vi "Calculator.vi"() -> ()   [LabVIEW 2015]
panel:
  out "Display":string
  out "Numeric 2":dbl
  out "Numeric":dbl format="%#_9g"
  out "Operator":string
  in  "N":dbl=1.0
  in  "Boolean":bool
  in  "stop":bool
  in  "8":bool
  in  "=":bool
  in  ".":bool
  in  "+":bool
  in  "3":bool
  in  "0":bool
  in  "Negative":bool
  in  "2":bool
  in  "1":bool
  in  "-":bool
  in  "6":bool
  in  "*":bool
  in  "9":bool
  in  "5":bool
  in  "4":bool
  in  "7":bool
  in  "\\":bool
  in  "C":bool
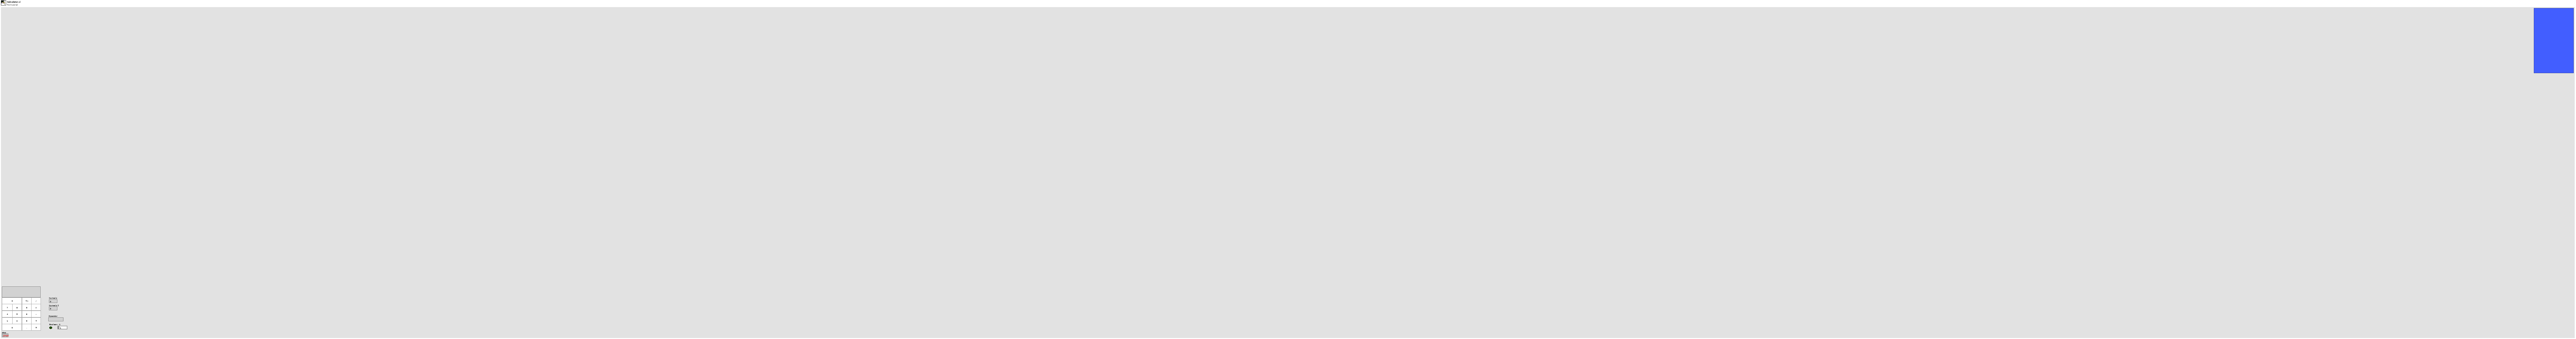
[diagram p1: front panel]
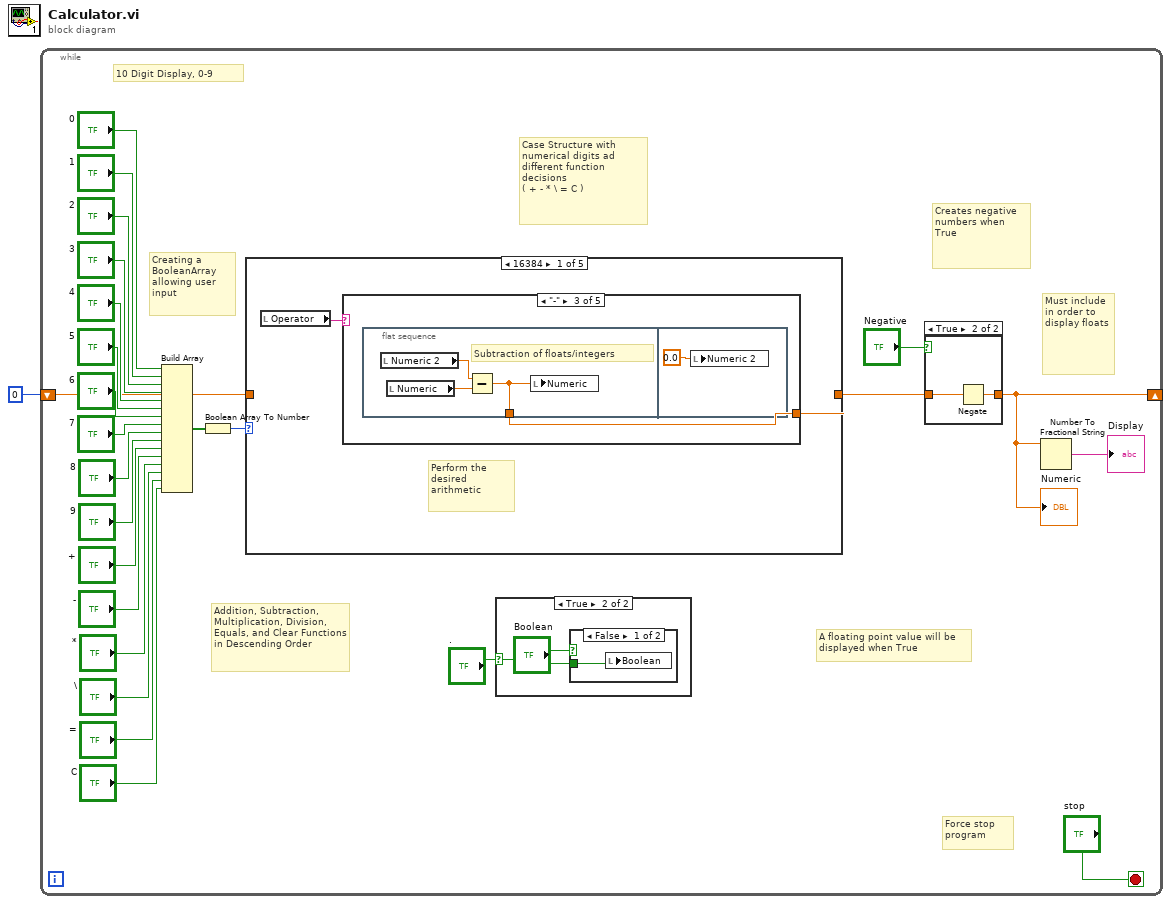
[diagram p0: block diagram]
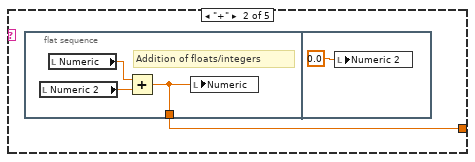
[diagram p6: hidden frame]
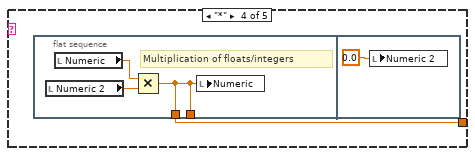
[diagram p7: hidden frame]
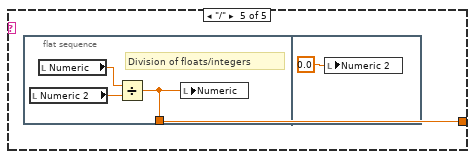
[diagram p8: hidden frame]
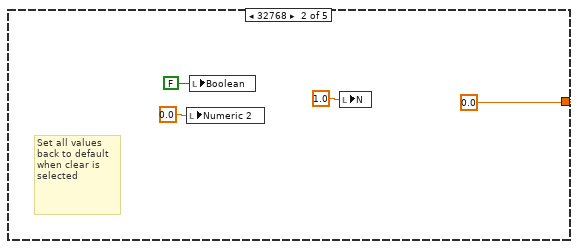
[diagram p9: hidden frame]
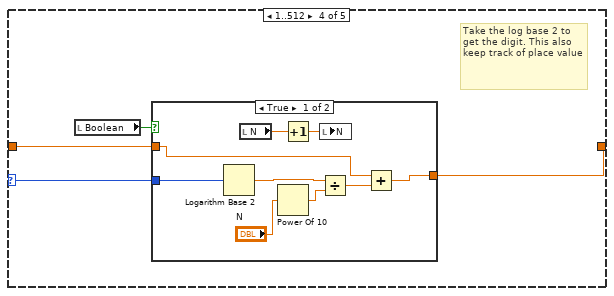
[diagram p11: hidden frame]
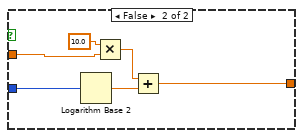
[diagram p12: hidden frame]
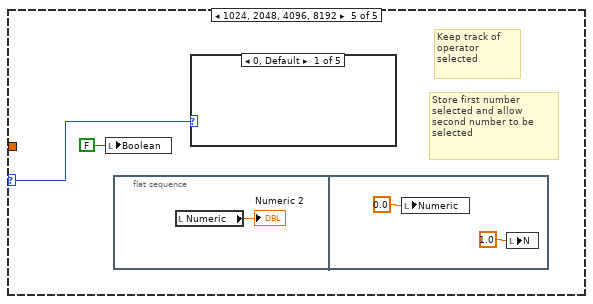
[diagram p13: hidden frame]
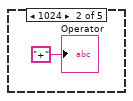
[diagram p14: hidden frame]
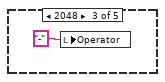
[diagram p15: hidden frame]
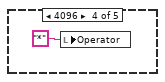
[diagram p16: hidden frame]
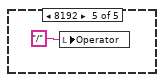
[diagram p17: hidden frame]
diagram:
  n1 = while {
    shift-right: [w3] -> _
    shift-left: 0 -> [w10]
    stop <- "stop" stop-if-true
    # "Force stop program"
    # "Must include in order to display floats"
    # "A floating point value will be displayed when True"
    # "Creates negative numbers when True"
    # "Case Structure with numerical digits ad different function decisions\n( + - * \\ = C )"
    # "Creating a BooleanArray allowing user input"
    # "Addition, Subtraction, Multiplication, Division, Equals, and Clear Functions in Descending Order"
    # "10 Digit Display, 0-9"
    n2 = Build Array("0", "1", "2", "3", "4", "5", "6", "7", "8", "9", "+", "-", "*", "\\", "=", "C") -> (w17:bool[])
    n3 = Boolean Array To Number(Boolean array=w17) -> (number=w9:u32)
    n4 = case shown="16384" w9 {
      selector: w9 -> [_ _ _ w63 w80]
      tunnel: w10 -> [_ _ w59 w61 _]
      tunnel: [w33 0.0 w59 w60 _] -> w4
      frame 16384 {
        # "Perform the\ndesired arithmetic"
        n5 = local read "Operator"() -> (w34:string)
        n6 = case shown="\"-\"" w34 {
          tunnel: [_ w35 w40 w45 w50] -> w33
          frame Default {
          }
          frame "+" {
            n7 = flat-sequence {
              tunnel: [w36] -> w35
              frame #0 {
                # "Addition of floats/integers"
                n8 = local read "Numeric 2"() -> (w37:dbl)
                n9 = local read "Numeric"() -> (w38:dbl)
                n10 = Add(x=w38, y=w37) -> (x+y=w36:dbl)
                n11 = local write "Numeric"(w36) -> ()
              }
              frame #1 {
                n12 = local write "Numeric 2"(0.0 ("Numeric 2")) -> ()
              }
            }
          }
          frame "-" {
            n13 = flat-sequence {
              tunnel: [w43] -> w40
              frame #0 {
                # "Subtraction of floats/integers"
                n14 = local read "Numeric 2"() -> (w42:dbl)
                n15 = local read "Numeric"() -> (w41:dbl)
                n16 = Subtract(x=w42, y=w41) -> (x-y=w43:dbl)
                n17 = local write "Numeric"(w43) -> ()
              }
              frame #1 {
                n18 = local write "Numeric 2"(0.0 ("Numeric 2")) -> ()
              }
            }
          }
          frame "*" {
            n19 = flat-sequence {
              tunnel: [w46] -> _
              tunnel: [w46] -> w45
              frame #0 {
                # "Multiplication of floats/integers"
                n20 = local read "Numeric 2"() -> (w47:dbl)
                n21 = local read "Numeric"() -> (w48:dbl)
                n22 = Multiply(x=w48, y=w47) -> (x*y=w46:dbl)
                n23 = local write "Numeric"(w46) -> ()
              }
              frame #1 {
                n24 = local write "Numeric 2"(0.0 ("Numeric 2")) -> ()
              }
            }
          }
          frame "/" {
            n25 = flat-sequence {
              tunnel: [w51] -> w50
              frame #0 {
                # "Division of floats/integers"
                n26 = local read "Numeric 2"() -> (w52:dbl)
                n27 = local read "Numeric"() -> (w53:dbl)
                n28 = Divide(x=w53, y=w52) -> (x/y=w51:dbl)
                n29 = local write "Numeric"(w51) -> ()
              }
              frame #1 {
                n30 = local write "Numeric 2"(0.0 ("Numeric 2")) -> ()
              }
            }
          }
        }
      }
      frame 32768 {
        # "Set all values back to default when clear is selected"
        n31 = local write "Numeric 2"(0.0 ("Numeric 2")) -> ()
        n32 = local write "Boolean"(FALSE ("Boolean")) -> ()
        n33 = local write "N"(1.0 ("N")) -> ()
      }
      frame 0, Default {
      }
      frame 1..512 {
        # "Take the log base 2 to get the digit. This also keep track of place value"
        n34 = local read "Boolean"() -> (w62:bool)
        n35 = case shown="True" w62 {
          tunnel: w63 -> [w72 w78]
          tunnel: w61 -> [w65 w77]
          tunnel: [w64 w73] -> w60
          frame True {
            n36 = Logarithm Base 2(1:w72) -> (0:w68:dbl)
            n37 = local read "N"() -> (w71:dbl)
            n38 = Power Of 10(x="N") -> (10^x=w67:dbl)
            n39 = Increment(x=w71) -> (x+1=w70:dbl)
            n40 = local write "N"(w70) -> ()
            n41 = Divide(x=w68, y=w67) -> (x/y=w66:dbl)
            n42 = Add(x=w65, y=w66) -> (x+y=w64:dbl)
          }
          frame False {
            n43 = Logarithm Base 2(1:w78) -> (0:w74:dbl)
            n44 = Multiply(x=10.0, y=w77) -> (x*y=w75:dbl)
            n45 = Add(x=w75, y=w74) -> (x+y=w73:dbl)
          }
        }
      }
      frame 1024, 2048, 4096, 8192 {
        # "Store first number selected and allow second number to be selected"
        # "Keep track of operator selected"
        n46 = local write "Boolean"(FALSE ("Boolean")) -> ()
        n47 = flat-sequence {
          frame #0 {
            n48 = local read "Numeric"() -> (→"Numeric 2":dbl)
          }
          frame #1 {
            n49 = local write "Numeric"(0.0 ("Numeric")) -> ()
            n50 = local write "N"(1.0 ("N")) -> ()
          }
        }
        n51 = case shown="0, Default" w80 {
          frame 0, Default {
          }
          frame 1024 {
            "Operator" <- "+" ("String")
          }
          frame 2048 {
            n52 = local write "Operator"("-" ("String")) -> ()
          }
          frame 4096 {
            n53 = local write "Operator"("*" ("String")) -> ()
          }
          frame 8192 {
            n54 = local write "Operator"("/" ("String")) -> ()
          }
        }
      }
    }
    n55 = case shown="True" "." {
      selector: "." -> [_ w31]
      frame False {
      }
      frame True {
        n56 = case shown="False" "Boolean" {
          tunnel: w31 -> [w32 _]
          frame False {
            n57 = local write "Boolean"(w32) -> ()
          }
          frame True {
          }
        }
      }
    }
    n58 = case shown="True" "Negative" {
      tunnel: w4 -> [w27 w29]
      tunnel: [w27 w28] -> w3
      frame False {
      }
      frame True {
        n59 = Negate(x=w29) -> (-x=w28:dbl)
      }
    }
    "Numeric" <- w3
    n60 = Number To Fractional String(number=w3) -> (F-format string=→"Display":string)  [unwired: 3 in]
  }
